vi "串口配置.vi"(8 "PORT":string="1001", 9 "IP":string="127.0.0.1", 10 "MB通信方式选择":enum16{"串口", "TCP"}(ring), 11 "请选择串口:":refnum<visa-resource-name>) -> (0 "PORT 2":string="1001", 1 "IP 2":string="127.0.0.1", 2 "确认 2":bool, 3 "VISA资源名称 2":refnum<visa-resource-name>, 4 "MB通信方式选择 2":enum16{"串口", "TCP"}(ring))   [LabVIEW 2016, in "德润DR803L超标留样.lvlib"]
panel:
  in  "取消":bool
  in  "确认":bool
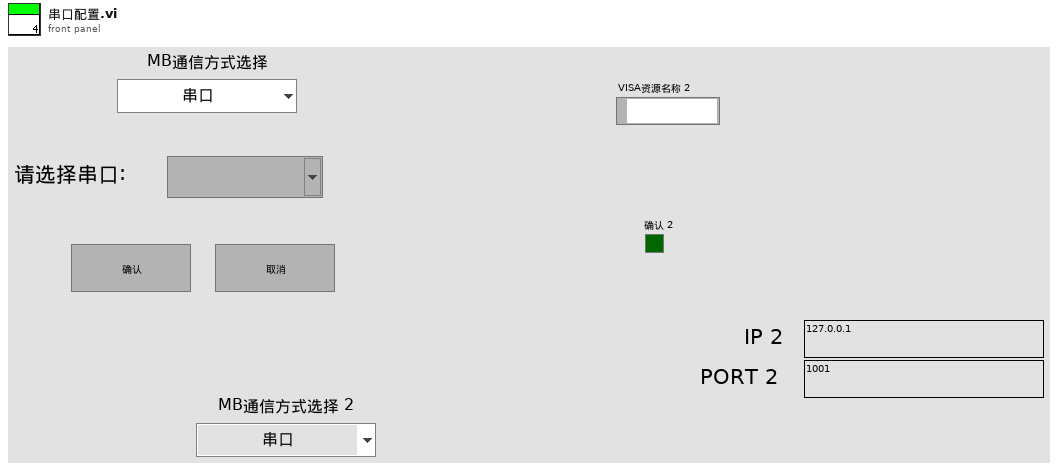
[diagram p1: front panel]
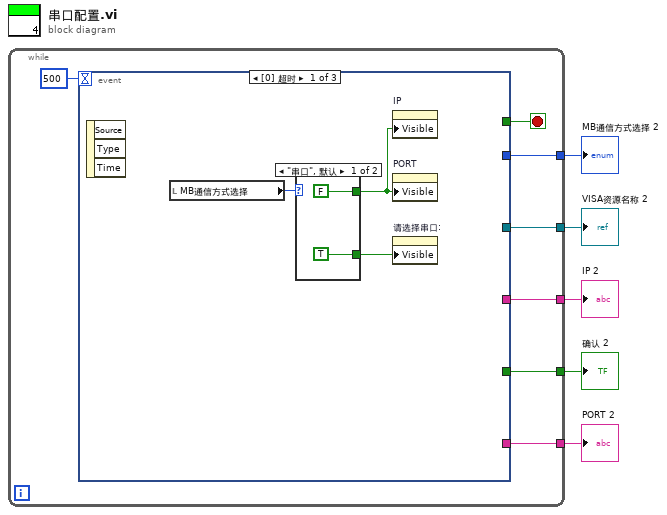
[diagram p0: block diagram]
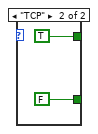
[diagram p2: hidden frame]
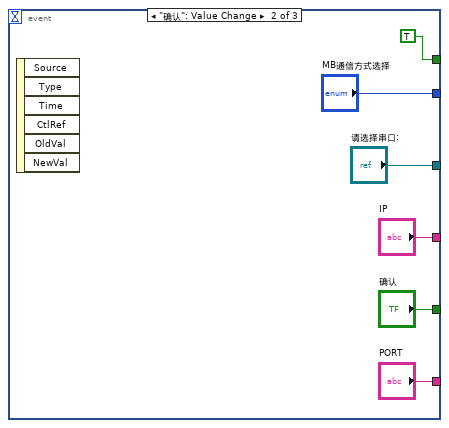
[diagram p3: hidden frame]
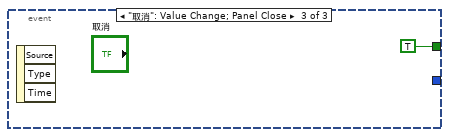
[diagram p4: hidden frame]
diagram:
  n1 = while {
    tunnel: [w12] -> w5
    tunnel: [w10] -> w4
    tunnel: [w9] -> w3
    tunnel: [w8] -> w2
    tunnel: [w7] -> w1
    stop <- w11 stop-if-true
    n2 = event shown="[0] 超时" {
      selector: _ -> [_ _ _]
      dyn-events: _ -> [_ _ _]
      timeout: 500 -> [_ _ _]
      tunnel: [_ "请选择串口:" _] -> w12
      tunnel: [_ TRUE TRUE] -> w11
      tunnel: [_ "确认" _] -> w10
      tunnel: [_ "IP" _] -> w9
      tunnel: [_ "PORT" _] -> w8
      tunnel: [_ "MB通信方式选择" _] -> w7
      event Timeout {
        n3 = event-data() -> ()  [unwired: 1 in, 3 out]
        n4 = local read "MB通信方式选择"() -> (w13:enum16{"串口", "TCP"})
        n5 = case shown="\"串口\", 默认" w13 {
          tunnel: [FALSE ("可见") TRUE ("可见")] -> w14
          tunnel: [TRUE ("可见") FALSE ("可见")] -> w15
          frame "串口", Default {
          }
          frame "TCP" {
          }
        }
        n6 = property on="IP" class="Str"("Visible"=w14) -> ()  [unwired: 2 in, 2 out]
        n7 = property on="PORT" class="Str"("Visible"=w14) -> ()  [unwired: 2 in, 2 out]
        n8 = property on="请选择串口:" class="VISAName"("Visible"=w15) -> ()  [unwired: 2 in, 2 out]
      }
      event "确认": Value Change {
        n9 = event-data() -> ()  [unwired: 1 in, 6 out]
      }
      event "取消": Value Change; Panel Close {
        n10 = event-data() -> ()  [unwired: 1 in, 3 out]
      }
    }
  }
  "VISA资源名称 2" <- w5
  "确认 2" <- w4
  "IP 2" <- w3
  "PORT 2" <- w2
  "MB通信方式选择 2" <- w1
